vi "Pre Launch Init.vi"(11 "Generic Optimization in":refnum<class "Generic Optimization.lvclass">) -> (0 "error out":errorcluster, 3 "Generic Optimization out":refnum<class "Generic Optimization.lvclass">)   [LabVIEW 2018, in "Generic Optimization Actor.lvlib" / "Generic Optimization.lvclass"]
doc: "(<B>Filename</B>: Actor Framework.lvlib:Actor.lvclass:Pre Launch Init.vi)\n\nDefines behavior that occurs after the Launch Nested Actor method is invoked but before the actor's Actor Core method begins running.\n\nBy default, this method does nothing. A descendant class may override it to define behavior."
uses:
  Generic Optimization.lvclass
  C:/Program Files (x86)/National Instruments/LabVIEW 2018/vi.lib/ActorFramework/Actor/Actor.lvclass
  C:/Users/Administrator/Desktop/2018LabVIEW EMS/Device Communication and Control Abstract Actor/Device Communication and Control Abstract/Device Communication and Control Abstract.lvclass
  <vilib>/ActorFramework/Actor/Actor.lvclass/Actor.ctl
  Device Communication and Control Abstract Actor/Device Communication and Control Abstract/Device Communication and Control Abstract.lvclass/Device Communication and Control Abstract.ctl
  Generic Optimization.lvclass/Generic Optimization.ctl
  Device Communication and Control Abstract Actor/Device Communication and Control Abstract Messages/Set IED watchdogReset Msg/Set IED watchdogReset Msg.lvclass
  C:/Program Files (x86)/National Instruments/LabVIEW 2018/vi.lib/ActorFramework/Message/Message.lvclass
  Device Communication and Control Abstract Actor/Device Communication and Control Abstract/Device Communication and Control Abstract.lvclass
  <vilib>/ActorFramework/Actor/Actor.lvclass
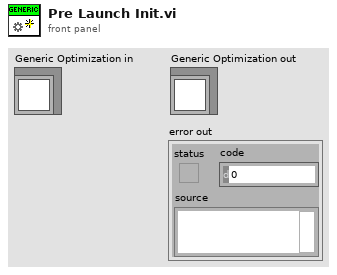
[diagram p1: front panel]
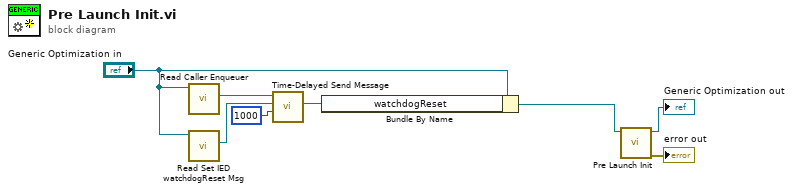
[diagram p0: block diagram]
diagram:
  n1 = call <vilib>:"Read Caller Enqueuer.vi"("Actor"="Generic Optimization in") -> ("Caller Enqueuer"=w5:refnum<class "Message Enqueuer.lvclass">)  [unwired: 10 in]
  n2 = call "Read Set IED watchdogReset Msg.vi"("SCADA Sub Abstract in"="Generic Optimization in") -> ("Set IED watchdogReset Msg"=w4:refnum<class "Set IED watchdogReset Msg.lvclass">)  [unwired: 9 in, 1 out]
  n3 = call <vilib>:"Time-Delayed Send Message.vi"("Milliseconds To Wait"=1000, "Message"=w4, "Message Enqueuer"=w5) -> ("Delivery Notifier"=w1:refnum<notifier>)  [unwired: 7 in, 1 out]
  n4 = Bundle By Name(cluster="Generic Optimization in", "watchdogReset"=w1) -> (w2:refnum<class "Generic Optimization.lvclass">)
  n5 = call-parent "Pre Launch Init.vi"("EMS Generic in"=w2) -> ("error out"=→"error out":errorcluster, "EMS Generic out"=→"Generic Optimization out":refnum<class "Generic Optimization.lvclass">)  [unwired: 9 in]
